vi "n set ext start delay.vi"(8 "error in (no error)":errorcluster, 9 "encoder":i16, 10 "delay":i16, 11 "n":u16) -> (0 "error out":errorcluster)   [LabVIEW 2015, in "SCANalone4x64.lvlib"]
doc: "__declspec(dllimport) void __stdcall n_set_ext_start_delay(unsigned short n, short delay, short encoder);"
uses:
  <userlib>/SCANalone4x64/SCANalone4x64.lvlib
  <userlib>/SCANalone4x64/SCANalone4x64.dll
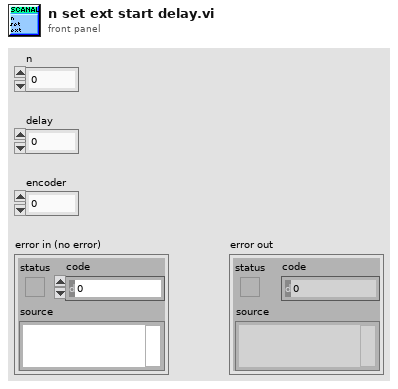
[diagram p1: front panel]
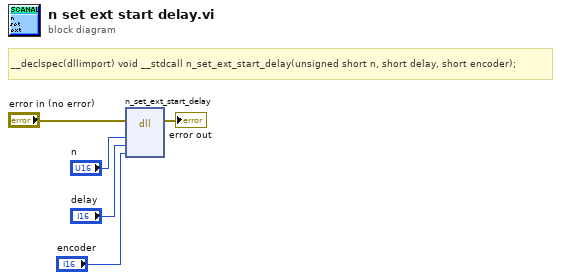
[diagram p0: block diagram]
diagram:
  # "__declspec(dllimport) void __stdcall n_set_ext_start_delay(unsigned short n, short delay, short encoder);"
  n1 = dll-call lib="C:/Program Files/National Instruments/LabVIEW 2015/user.lib/SCANalone4x64/SCANalone4x64.*" fn="n_set_ext_start_delay"(error in="error in (no error)", "n"="n", "delay"="delay", "encoder"="encoder") -> (error out=→"error out":errorcluster)  [unwired: 6 in, 1 out]
